vi "Process Lidar Data.vi"(6 "Estimated Pose After Scan":cluster{"X":dbl, "Y":dbl, "R":dbl}, 7 "Estimated Pose Before Scan":cluster{"X":dbl, "Y":dbl, "R":dbl}, 9 "Direction":dbl[](array[numeric]), 10 "Magnitude":dbl[](array[numeric]), 11 "path in":path) -> (2 "Data Comparison":cluster{"X":dbl[], "Y":dbl[]}[](array[cluster]), 3 "Lidar Scan":T1)   [LabVIEW 2017]
uses:
  control/Robot Properties.vi
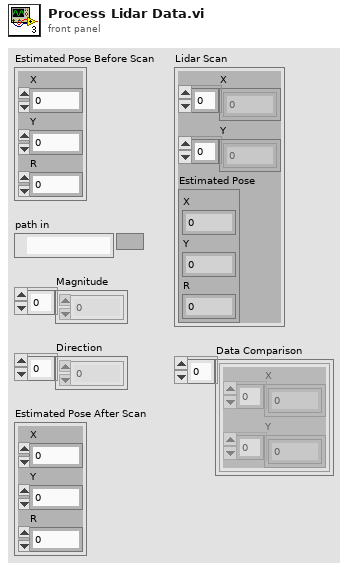
[diagram p1: front panel]
types:
  T1 = cluster{"X":dbl[], "Y":dbl[], "Estimated Pose":cluster{"X":dbl, "Y":dbl, "R":dbl}}
  T2 = cluster{dbl[], dbl[], "Estimated Pose After Scan":cluster{"X":dbl, "Y":dbl, "R":dbl}}
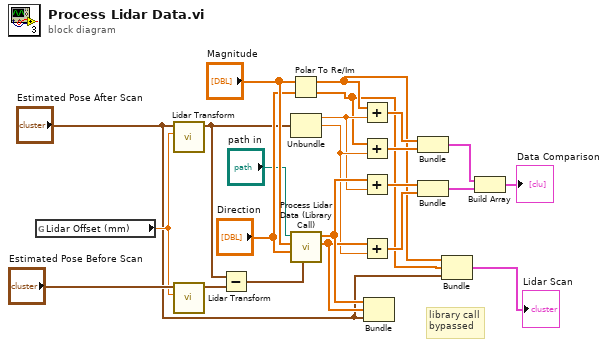
[diagram p0: block diagram]
diagram:
  # "library call\nbypassed"
  n1 = global read "Robot Properties.vi" "Lidar Offset (mm)"() -> (w5:dbl)
  n2 = call "Lidar Transform.vi"("Transform Amount (mm)"=w5, "Pose"="Estimated Pose After Scan") -> ("Pose"=w6:cluster{"X":dbl, "Y":dbl, "R":dbl})  [unwired: 9 in]
  n3 = call "Lidar Transform.vi"("Transform Amount (mm)"=w5, "Pose"="Estimated Pose Before Scan") -> ("Pose"=w17:cluster{"X":dbl, "Y":dbl, "R":dbl})  [unwired: 9 in]
  n4 = Subtract(x=w6, y=w17) -> (x-y=w19:cluster{"X":dbl, "Y":dbl, "R":dbl})
  n5 = Polar To Re/Im(2:"Direction", 3:"Magnitude") -> (0:w2:dbl[], 1:w3:dbl[])
  n6 = Unbundle(w6) -> ("X"=w9:dbl, "Y"=w10:dbl)  [unwired: 1 out]
  n7 = call "Process Lidar Data (Library Call).vi"("Pose Delta"=w19, "Direction"="Direction", "Magnitude"="Magnitude", "Library Path"="path in") -> ("Y"=w11:dbl[], "X"=w12:dbl[])  [unwired: 6 in]
  n8 = Add(x=w3, y=w9) -> (x+y=w14:dbl[])
  n9 = Add(x=w2, y=w10) -> (x+y=w13:dbl[])
  n10 = Add(x=w12, y=w9) -> (x+y=w8:dbl[])
  n11 = Add(x=w11, y=w10) -> (x+y=w7:dbl[])
  n12 = Bundle("X"=w12, "Y"=w11, "Estimated Pose After Scan"="Estimated Pose After Scan") -> ()  [unwired: 1 in, 1 out]
  n13 = Bundle(w14, w13) -> (w16:cluster{dbl[], dbl[]})  [unwired: 1 in]
  n14 = Bundle(w8, w7) -> (w15:cluster{dbl[], dbl[]})  [unwired: 1 in]
  n15 = Bundle(w3, w2, "Estimated Pose After Scan"="Estimated Pose After Scan") -> (→"Lidar Scan":T2)  [unwired: 1 in]
  n16 = Build Array(w16, w15) -> (→"Data Comparison":cluster{dbl[], dbl[]}[])
